vi "字符串转数学公式.vi"() -> ()   [LabVIEW 2023]
uses:
  <vilib>/express/express arith-compare/Formula/XNode/ExpressFormulaBlockNode.xnode
  <vilib>/gmath/NI_Gmath.lvlib
panel:
  out "Result":dbl
  in  "X2":dbl
  in  "X1":dbl
  out "y value":dbl format="%.2f"
  in  "formula":string
  # "字符串转数学公式 - 3"
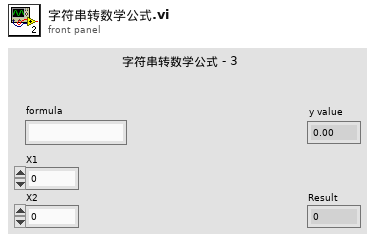
[diagram p1: front panel]
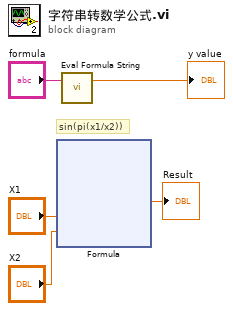
[diagram p0: block diagram]
diagram:
  # "sin(pi(x1/x2))"
  n1 = xnode "Formula"("X1"="X1", "X2"="X2") -> ("Result"=→"Result":dbl)  [unwired: 1 in, 1 out]
  n2 = call <vilib>:"Eval Formula String.vi"("formula"="formula") -> ("y value"=→"y value":dbl)  [unwired: 1 in, 1 out]
